vi "MotorTuning.vi"() -> ()   [LabVIEW 2017]
uses:
  <vilib>/Platform/TimedLoop/XDataNode/wakeup.ctl
  <vilib>/Platform/TimedLoop/XDataNode/XDNodeRunTimeDep.lvlib
  <vilib>/Platform/TimedLoop/XDataNode/nitl_modes.ctl
  <vilib>/Platform/TimedLoop/XDataNode/timing_clust.ctl
  <vilib>/Platform/TimedLoop/XDataNode/XDataNode.xnode
  <vilib>/addons/control/pid/NI_PID_pid.lvlib
  <vilib>/addons/control/pid/pid.llb/PID Output Rate Limiter (DBL Array).vi
  typeDef/Modes.ctl
  <vilib>/rvi/interface/nirviReadWriteControl/nirviReadWriteControl.xnode
  <vilib>/Utility/error.llb/Error Cluster From Error Code.vi
  <vilib>/rvi/interface/Simulation/niFpgaSimulationCallBeginRW.vi
  <vilib>/rvi/errors/niLvFpgaAdjustHostInterfaceError.vi
  NiFpgaLv.dll
  subVIs_target/GlobalVariables.vi
  <vilib>/addons/control/pid/pid.llb/PID (DBL).vi
panel:
  in  "?":string="PID_M1.txt"
  in  "FF only once":bool=TRUE
  out "noiseCT":dbl
  in  "amp and freq":dbl[](array[numeric])=[0.0, 0.0, 0.0, 0.0]
  out "nS":dbl
  in  "Noise":bool
  out "dWrite":dbl[](array[numeric])
  in  "filtLowCutFreq":dbl=10.0
  in  "filtOrder":i32=2
  in  "PID_betas":dbl[](array[numeric])=[1.0]
  in  "Mag (N)":dbl=20.0
  in  "Force":bool
  in  "PID gains":T1(array[cluster])=[{"proportional gain (Kc)"=3.5, "integral time (Ti, min)"=0.001, "derivative time (Td, min)"=0.0004}]
  in  "?":bool
  in  "Motor No":i32
  out "currentTension":dbl
  out "whichMotors":i32[](array[numeric])
  out "nMotors":i32
  out "ff+fb OP (N)":dbl[](array[numeric])
  out "setTension":dbl
  out "Period":dbl
  in  "PID_OP_upLim":dbl=60.0
  out "frictionV":dbl[](array[numeric])
  out "CableReelAng(deg)":dbl[](array[numeric])
  out "refnum out":refnum<file>
  in  "Record":bool
  in  "SetPt loop period":i64=4000
  in  "Voltage":dbl(slide) scale=0.0..2.5
  in  "Stop":bool
  in  "pidLpPrd":i64=1000
  in  "Manual":bool
  out "FFnFB OP (N)":dbl[](array[numeric])
  out "Voltage O/P (V)":dbl[](graph)
  out "?":T2(graph)
  in  "?":bool
  in  "freq and step":dbl[](array[numeric])=[0.0, 0.0, 0.0, 0.0]
  in  "Constant":bool
  in  "Idle":bool
  in  "LoadCell No":i32
  out "OP (V)":dbl[](array[numeric])
  out "Iteration Duration":i64
  out "Iteration Duration 2":i64
  # "Amp (N)\n\nfreq (Hz)\n\nSTEP (N)"
  # "Desired (N)"
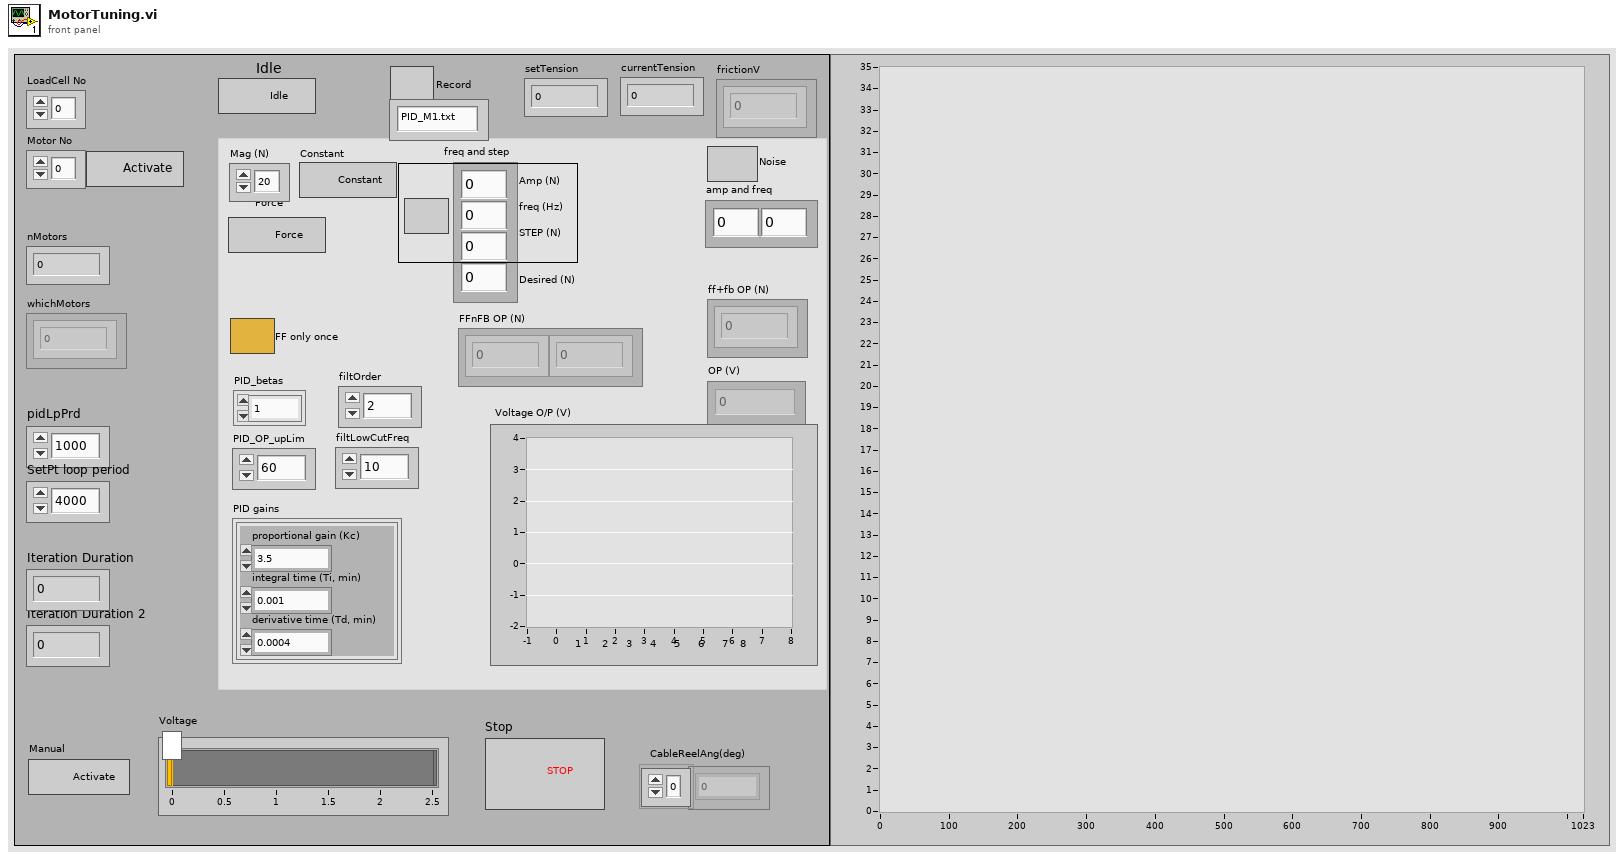
[diagram p1: front panel]
types:
  T1 = cluster{"proportional gain (Kc)":dbl, "integral time (Ti, min)":dbl, "derivative time (Td, min)":dbl}[]
  T2 = cluster{"[0]":dbl, "[1]":dbl, "[2]":dbl, "[3]":dbl, "[4]":dbl, "[5]":dbl, "[6]":dbl, "[7]":dbl}
  T3 = typedef "Modes.ctl" = enum16{"Idle", "Constant", "Force", "Pert"}
  T4 = enum16{"open", "replace", "create", "open or create", "replace or create", "replace or create with confirmation"}
  T5 = typedef "XDNodeRunTimeDep.lvlib/timing_clust.ctl" = cluster{"Expected End [f-1]":u64, "Actual End [f-1]":u64, "Finished Late? [f-1]":bool, "Expected End [i-1]":u64, "Actual End [i-1]":u64, "Finished Late? [i-1]":bool, "Expected Start [i]":u64, "Actual Start [i]":u64, "Expected Start [f]":u64, "Actual Start [f]":u64, "Source Name":string, "Structure Name":string, "Period":i64, "Deadline":i64, "Offset":i64, "Start":i64, "Priority":i32, "Timeout":i32, "Mode":T6, "Wakeup Reason":T7, "Error":errorcluster, "Source Type":string, "Secondary Source Type":string, "Global End Time":u64, "Global Start Time":u64, "Frame Duration":u64, "Iteration Duration":u64, "Assigned CPU":i32, "I/O Scan Engine Mode":u32}
  T6 = typedef "XDNodeRunTimeDep.lvlib/nitl_modes.ctl" = enum32{"No Change", "Process missed periods, maintain original phase", "Discard missed periods, maintain original phase", "Process missed periods, ignore original phase", "Discard missed periods, ignore original phase"}
  T7 = typedef "XDNodeRunTimeDep.lvlib/wakeup.ctl" = enum32{"Normal", "Aborted", "Asynchronous wakeup", "Timing source error", "Timed loop error", "Timeout"}
  T8 = cluster{"fsp":dbl, "fvp":dbl, "fsn":dbl, "fvn":dbl}[]
  T9 = typedef "constants_LL.ctl" = cluster{"zero array":dbl[], "decRate_ff":dbl[], "Motor constants":dbl[], "PID gains":cluster{"proportional gain (Kc)":dbl, "integral time (Ti, min)":dbl, "derivative time (Td, min)":dbl}[], "decRate _fb":dbl[], "PID_OP_upLim":dbl, "nMotors":i32, "PID_betas":dbl[], "filtOrder":i32, "filtLowCutFreq":dbl, "filtSamplFreq":dbl, "whichMotors":i32[], "nMotors 1":i32, "nMotors 2":i32, "Motor constants pel":dbl[], "Motor constants trunk":dbl[]}
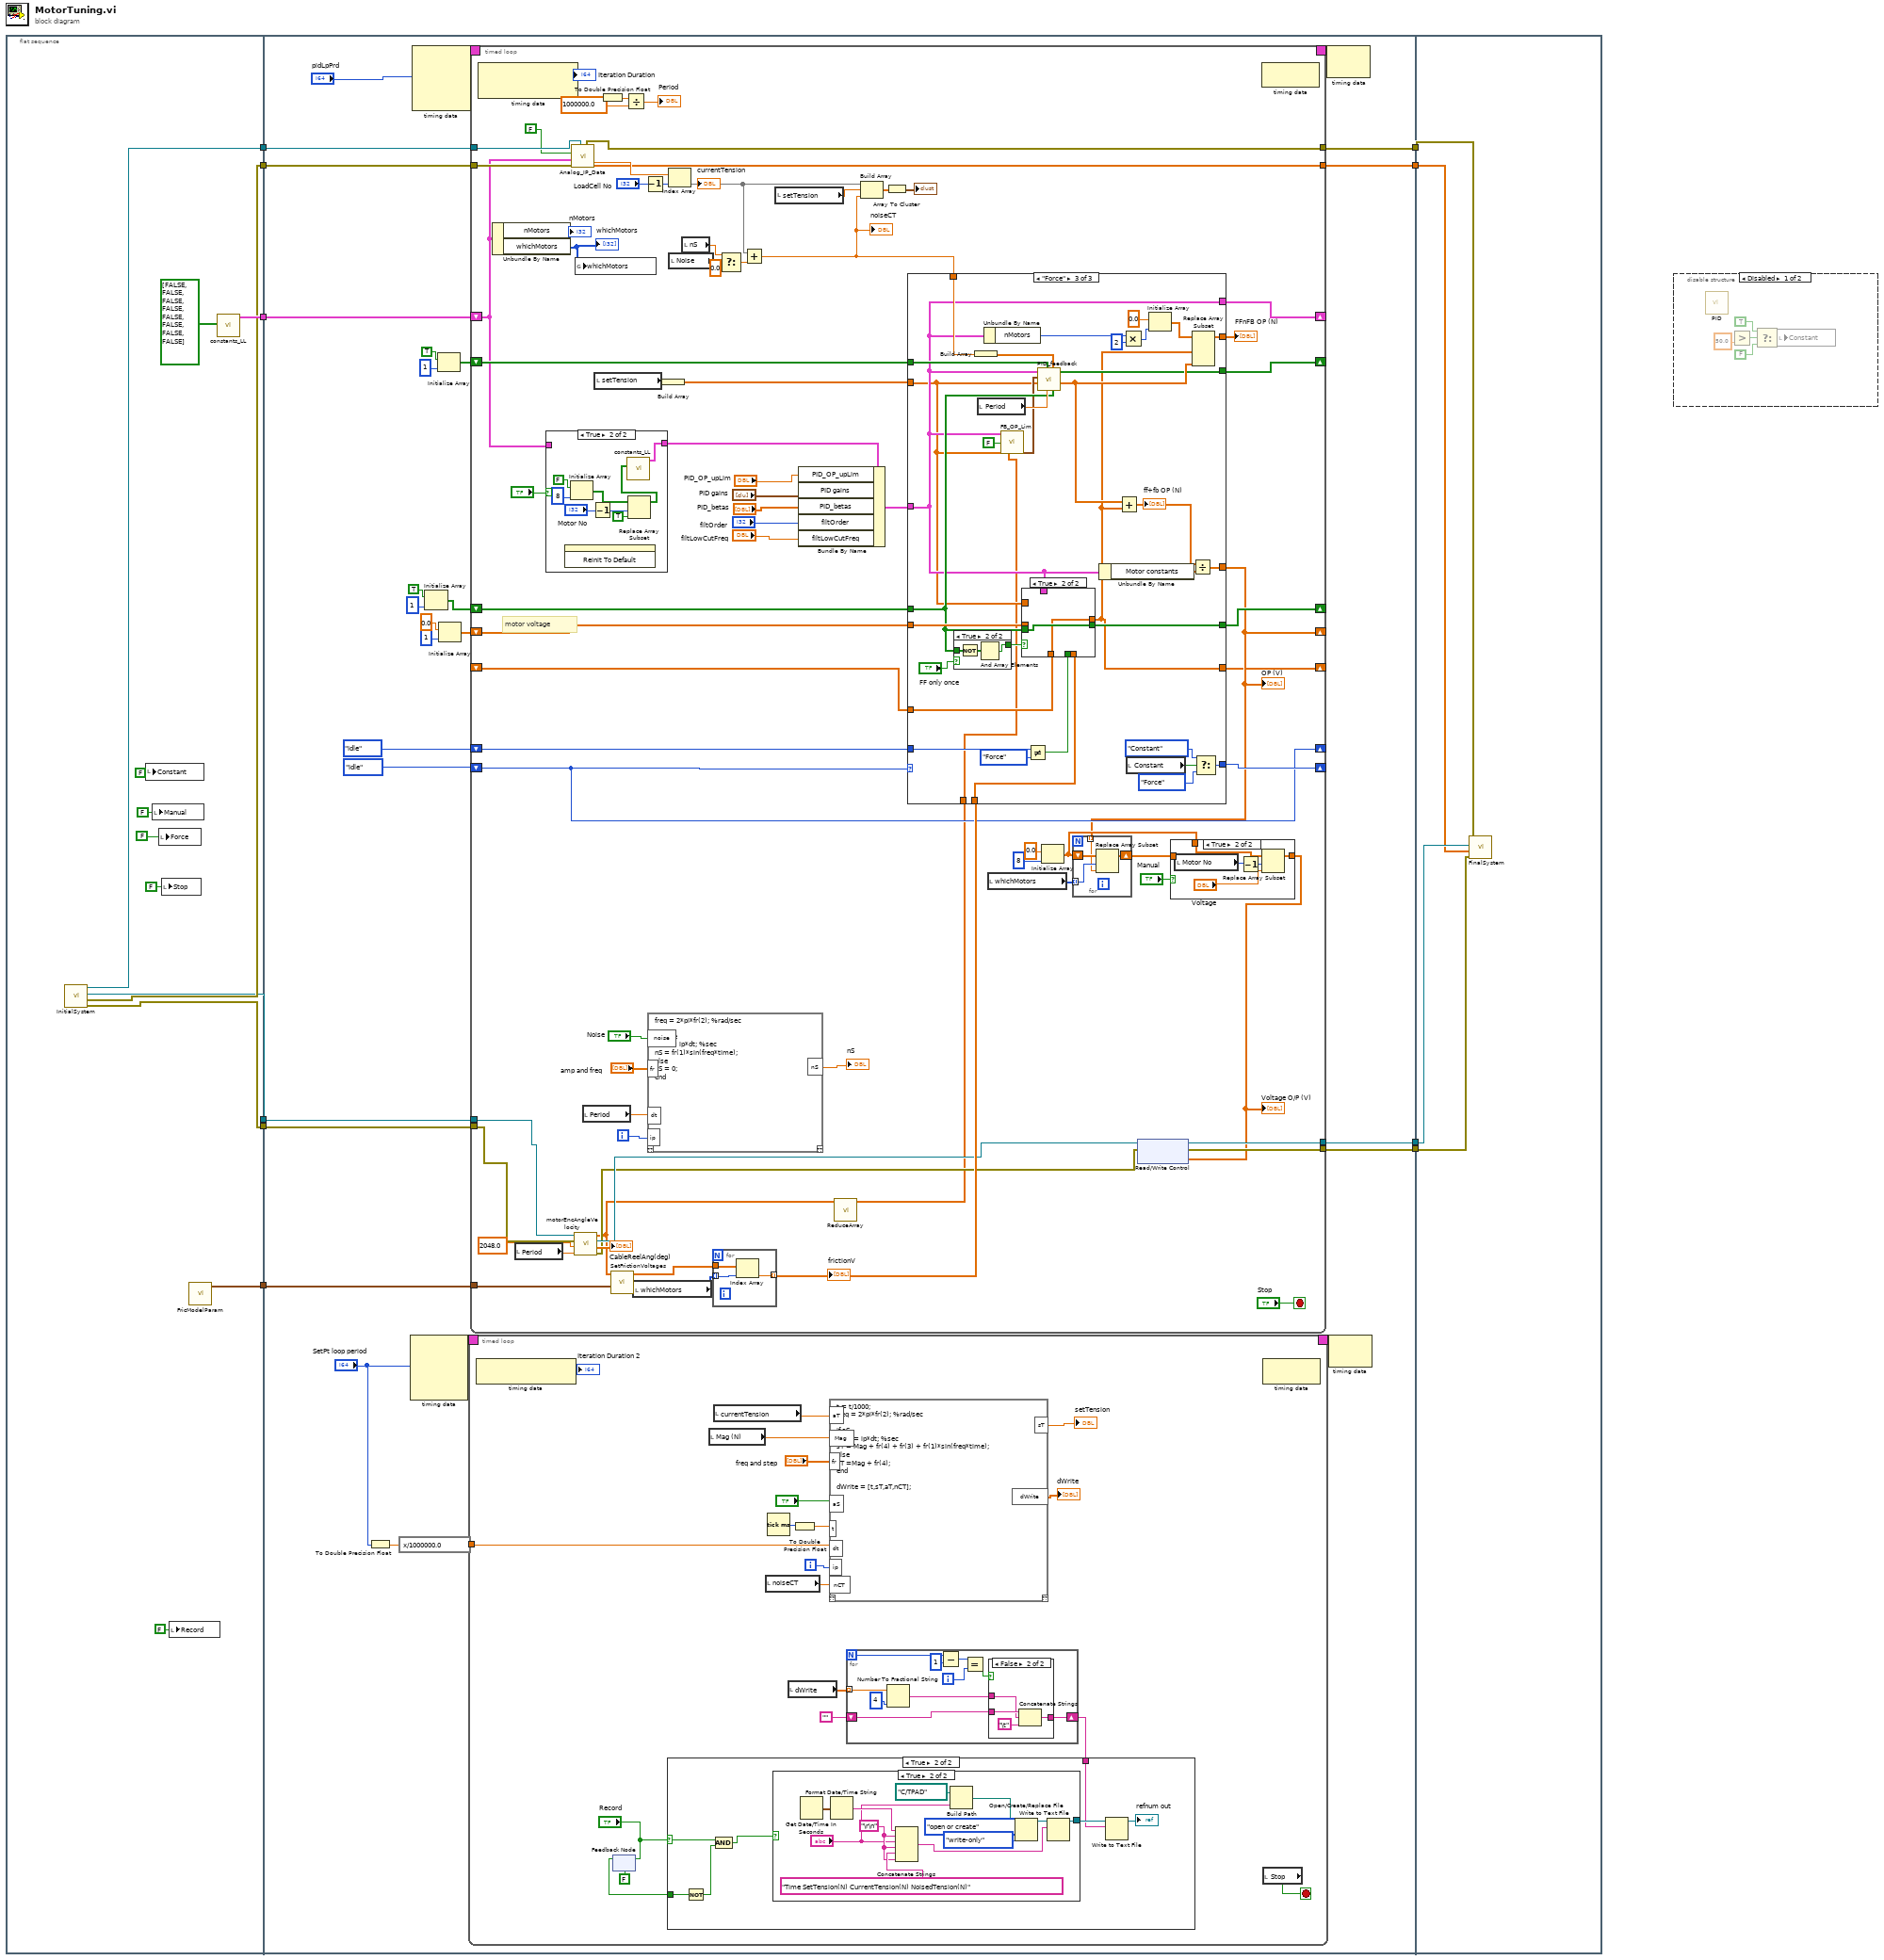
[diagram p0: block diagram]
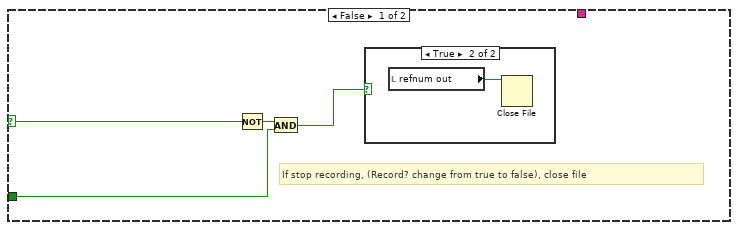
[diagram p3: hidden frame]
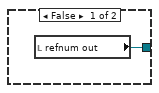
[diagram p5: hidden frame]
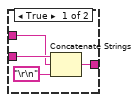
[diagram p6: hidden frame]
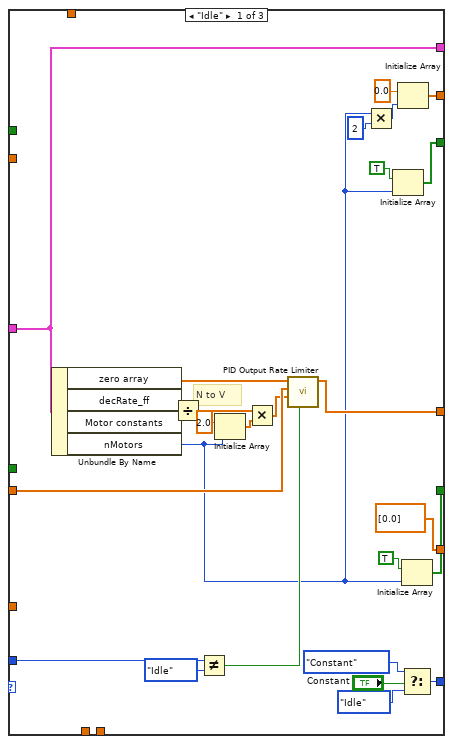
[diagram p9: hidden frame]
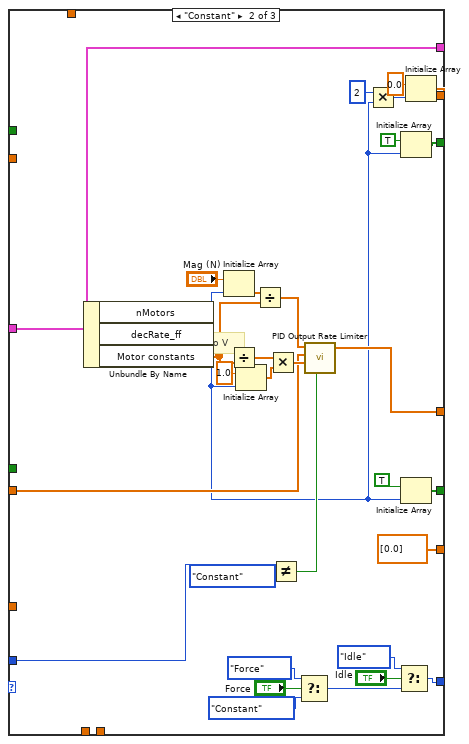
[diagram p10: hidden frame]
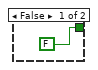
[diagram p11: hidden frame]
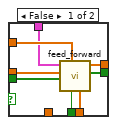
[diagram p12: hidden frame]
diagram:
  n1 = flat-sequence {
    tunnel: [w14] -> w10
    tunnel: [w12] -> w9
    tunnel: [w22] -> w8
    tunnel: [w21] -> w7
    tunnel: [w11] -> w5
    tunnel: [w13] -> w4
    tunnel: w10 -> [w47]
    tunnel: [w46] -> w6
    tunnel: w9 -> [w45]
    tunnel: w8 -> [w44]
    tunnel: w7 -> [w43]
    tunnel: w5 -> [w27]
    tunnel: w4 -> [w26]
    tunnel: [w25] -> w3
    tunnel: [w24] -> w2
    tunnel: [w23] -> w1
    tunnel: w6 -> [w335]
    tunnel: w3 -> [w338]
    tunnel: w2 -> [w337]
    tunnel: w1 -> [w336]
    frame #0 {
      n2 = call "InitialSystem.vi"() -> ("error out"=w13:errorcluster, "error out 2"=w12:errorcluster, "FPGA VI Reference Out"=w11:refnum<k20>, "Refnum out"=w14:refnum<k21>)  [unwired: 8 in]
      n3 = local write "Constant"(FALSE ("Force")) -> ()
      n4 = local write "Manual"(FALSE ("Manual")) -> ()
      n5 = local write "Force"(FALSE ("Force")) -> ()
      n6 = local write "Stop"(FALSE ("Stop")) -> ()
      n7 = local write "Record"(FALSE ("Record")) -> ()
      n8 = call "FricModelParam.vi"() -> ("FricModelParam"=w21:T8)  [unwired: 11 in]
      n9 = call "constants_LL.vi"("MotorsInUse"=bool[] [FALSE, FALSE, FALSE, FALSE, FALSE, FALSE, FALSE, FALSE] ("Enable Motors")) -> ("Constants LL"=w22:T9)  [unwired: 10 in]
    }
    frame #1 {
      n10 = To Double Precision Float(number="SetPt loop period") -> (double precision float=w37:dbl)
      n11 = expression code="x/1000000.0"(w37) -> (w39:dbl)
      n12 = node-c288("SetPt loop period") -> (w49:T5)  [unwired: 3 in]
      n13 = node-c288("pidLpPrd") -> (w51:T5)  [unwired: 3 in]
      n14 = Initialize Array(TRUE, 1 ("dimension size")) -> (w31:bool[])
      n15 = Initialize Array(TRUE, 1 ("dimension size")) -> (w30:bool[])
      n16 = Initialize Array(0.0 ("element"), 1 ("dimension size")) -> (w36:dbl[])
      n17 = timed-loop {
        timing: w49 -> [_]
        timing-out: [_] -> w48
        tunnel: w39 -> [w66]
        i -> [w58]
        stop <- w67 stop-if-true
        n18 = node-c288() -> (→"Iteration Duration 2":i64)  [unwired: 1 in]
        n19 = feedback-in #1("Record") -> ()
        n20 = feedback #1(FALSE) -> (w61:bool)
        n21 = local read "Mag (N)"() -> (w55:dbl)
        n22 = local read "currentTension"() -> (w56:dbl)
        n23 = local read "noiseCT"() -> (w52:dbl)
        n24 = Tick Count (ms)() -> (millisecond timer value=w70:u32)
        n25 = local read "dWrite"() -> (w53:dbl[])
        n26 = To Double Precision Float(number=w70) -> (double precision float=w69:dbl)
        n27 = mathscript code="t = t/1000;\nfreq = 2*pi*fr(2); %rad/sec\n\nif aS\ntime = ip*dt; %sec\nsT = Mag + fr(4) + fr(3) + fr(1)*sin(freq*time);\nelse\nsT =Mag + fr(4);\nend\n\ndWrite = [t,sT,aT,nCT];"("aS"="?", "ip"=w58, "fr"="freq and step", "t"=w69, "aT"=w56, "dt"=w66, "Mag"=w55, "nCT"=w52) -> ("dWrite"=→"dWrite":dbl[], "sT"=→"setTension":dbl)  [unwired: 1 in, 1 out]
        n28 = for {
          N -> [w100]
          tunnel: w53 -> [w104] mode=indexing
          shift-right: [w103] -> w63
          shift-left: "" -> [w102]
          i -> [w97]
          n29 = Number To Fractional String(number=w104, precision (6)=i16 4) -> (F-format string=w101:string)  [unwired: 2 in]
          n30 = Subtract(x=w100, y=1) -> (x-y=w98:i32)
          n31 = Equal?(x=w98, y=w97) -> (x = y?=w96:bool)
          n32 = case shown="False" w96 {
            tunnel: [w109 w113] -> w103
            tunnel: w102 -> [w108 w112]
            tunnel: w101 -> [w107 w111]
            frame True {
              n33 = Concatenate Strings(w108, w107, "\r\n") -> (w109:string)
            }
            frame False {
              n34 = Concatenate Strings(w112, w111, "\t") -> (w113:string)
            }
          }
        }
        n35 = case shown="True" "Record" {
          selector: "Record" -> [w73 w76]
          tunnel: w63 -> [_ w81]
          tunnel: w61 -> [w72 w79]
          frame False {
            # "If stop recording, (Record? change from true to false), close file"
            n36 = Not(x=w73) -> (.not. x?=w74:bool)
            n37 = And(x=w74, y=w72) -> (x .and. y?=w71:bool)
            n38 = case shown="True" w71 {
              frame False {
              }
              frame True {
                n39 = local read "refnum out"() -> (w75:refnum<file>)
                n40 = Close File(refnum=w75) -> ()  [unwired: 1 in, 2 out]
              }
            }
          }
          frame True {
            n41 = Not(x=w79) -> (.not. x?=w78:bool)
            n42 = And(x=w76, y=w78) -> (x .and. y?=w77:bool)
            n43 = case shown="True" w77 {
              tunnel: [w83 w85] -> w82
              frame False {
                n44 = local read "refnum out"() -> (w83:refnum<file>)
              }
              frame True {
                w92 = "\r\n"
                n45 = Get Date/Time In Seconds() -> (seconds since 1Jan1904=w95:timestamp)
                n46 = Format Date/Time String(seconds (now)=w95) -> (date/time string=w94:string)  [unwired: 2 in]
                n47 = Concatenate Strings(w94, w92, "?", w92, "Time SetTension(N) CurrentTension(N) NoisedTension(N)", w92) -> (w86:string)
                n48 = Build Path(base path=path "C:/TPAD", name or relative path="?") -> (appended path=w90:path)
                n49 = Open/Create/Replace File(file path (use dialog)=w90, operation (0:open)=T4."open or create", access (0:read/write)=enum16{"read/write", "read-only", "write-only"}."write-only") -> (refnum out=w87:refnum<file>)  [unwired: 3 in, 2 out]
                n50 = Write to Text File(file (use dialog)=w87, text=w86) -> (refnum out=w85:refnum<file>)  [unwired: 2 in, 2 out]
              }
            }
            n51 = Write to Text File(file (use dialog)=w82, text=w81) -> (refnum out=→"refnum out":refnum<file>)  [unwired: 2 in, 2 out]
          }
        }
        n52 = node-c288() -> ()  [unwired: 1 in, 1 out]
        n53 = local read "Stop"() -> (w67:bool)
      }
      n54 = timed-loop {
        timing: w51 -> [_]
        timing-out: [_] -> w50
        tunnel: w47 -> [w135]
        tunnel: [w134] -> w46
        tunnel: w45 -> [w196]
        shift-right: [w158] -> _
        shift-left: Modes."Idle" ("Enum") -> [w195]
        shift-right: [w194] -> _
        shift-left: Modes."Idle" ("Enum") -> [w158]
        shift-right: [w157] -> _
        shift-left: w36 -> [w189]
        tunnel: w43 -> [w193]
        shift-right: [w191] -> _
        shift-left: w31 -> [w190]
        shift-right: [w183] -> _
        shift-left: w30 -> [w184]
        shift-right: [w165] -> _
        shift-left: w44 -> [w136]
        shift-right: [w149] -> _
        shift-left: _ -> [w148]
        tunnel: w27 -> [w129]
        tunnel: w26 -> [w128]
        tunnel: [w131] -> w25
        tunnel: [w130] -> w24
        tunnel: [w124] -> w23
        i -> [w141]
        stop <- "Stop" stop-if-true
        # "motor voltage"
        n55 = node-c288() -> (→"Iteration Duration":i64, w178:i64)  [unwired: 1 in]
        n56 = Unbundle By Name(w136) -> ("nMotors"=→"nMotors":i32, "whichMotors"=w122:i32[])
        "whichMotors" <- w122
        n57 = local read "Period"() -> (w176:dbl)
        n58 = case shown="True" "?" {
          tunnel: [w207 w210] -> w151
          tunnel: w136 -> [w207 _]
          frame False {
          }
          frame True {
            n59 = invoke class="Bool (strict)" method="Reinit To Default"() -> ()  [unwired: 3 in, 3 out]
            n60 = Initialize Array(FALSE, 8 ("dimension size")) -> (w213:bool[])
            n61 = Decrement(x="Motor No") -> (x-1=w208:i32)
            n62 = Replace Array Subset(array=w213, new element=TRUE ("new element/subarray"), index=w208) -> (w211:bool[])
            n63 = call "constants_LL.vi"("MotorsInUse"=w211) -> ("Constants LL"=w210:T9)  [unwired: 10 in]
          }
        }
        n64 = call "Analog_IP_Data.vi"("Refnum in"=w135, "error in (no error)"=w196, "Constants LL"=w136, "Use ATI"=FALSE ("ATI Connected")) -> ("Tared FT Reading"=w124:dbl[], "Toe"=w132:dbl, "error out"=w134:errorcluster)  [unwired: 1 in, 4 out]
        n65 = call "motorEncAngleVelocity.vi"("dt"=w176, "CPR"=2048.0, "error in (no error)"=w128, "Refnum in"=w129) -> ("error out"=w126:errorcluster, "CableReelPos(deg)"=→"CableReelAng(deg)":dbl[], "Refnum out"=w127:refnum<k20>, "CableReelVel(RPM)"=w123:dbl[])  [unwired: 4 in]
        n66 = global write "GlobalVariables.vi" "whichMotors"(w122) -> ()
        n67 = local read "Period"() -> (w138:dbl)
        n68 = local read "setTension"() -> (w173:dbl)
        n69 = To Double Precision Float(number=w178) -> (double precision float=w180:dbl)
        n70 = call "SetFrictionVoltages.vi"("FricModelParam"=w193, "EncoderVelocity(RPM)"=w123) -> ("FrictionVoltages"=w171:dbl[])  [unwired: 9 in]
        n71 = Divide(x=w180, y=1000000.0) -> (x/y=→"Period":dbl)
        n72 = local read "whichMotors"() -> (w170:i32[])
        n73 = Decrement(x="LoadCell No") -> (x-1=w166:i32)
        n74 = mathscript code="freq = 2*pi*fr(2); %rad/sec\n\nif noise\ntime = ip*dt; %sec\nnS = fr(1)*sin(freq*time);\nelse\nnS = 0;\nend"("ip"=w141, "noise"="Noise", "dt"=w138, "fr"="amp and freq") -> ("nS"=→"nS":dbl)  [unwired: 1 in, 1 out]
        n75 = Build Array(w173) -> (w174:dbl[])
        n76 = Index Array(array=w132, index=w166) -> (element=w143)
        "currentTension" <- w143
        n77 = local read "Noise"() -> (w147:bool)
        n78 = local read "nS"() -> (w146:dbl)
        n79 = for {
          tunnel: w170 -> [w217] mode=indexing
          tunnel: w171 -> [w218]
          tunnel: [w216] -> w169 mode=indexing
          n80 = Index Array(array=w218, index=w217) -> (element=w216:dbl)
        }
        "frictionV" <- w169
        n81 = Select(t=w146, s=w147, f=0.0) -> (s? t:f=w144:dbl)
        n82 = Add(x=w143, y=w144) -> (x+y=w142:dbl)
        "noiseCT" <- w142
        n83 = local read "setTension"() -> (w175:dbl)
        n84 = Bundle By Name(cluster=w151, "PID_OP_upLim"="PID_OP_upLim", "PID gains"="PID gains", "PID_betas"="PID_betas", "filtOrder"="filtOrder", "filtLowCutFreq"="filtLowCutFreq") -> (w150:T9)
        n85 = call "ReduceArray.vi"("I/P Array"=w123) -> ("Reduced Array"=w121:dbl[])  [unwired: 10 in]
        n86 = Build Array(w143, w175, w142) -> (w187:dbl[])
        n87 = Array To Cluster(array=w187) -> (cluster=→"?":T2)
        n88 = case shown="\"Force\"" w158 {
          tunnel: [w222 w273 w290] -> w194
          tunnel: w195 -> [w245 w271 w312]
          tunnel: [w238 w258 w303] -> w157
          tunnel: w189 -> [w243 w253 w309]
          tunnel: w142 -> [_ _ w285]
          tunnel: w169 -> [_ _ w299]
          tunnel: [w231 w257 w300] -> w191
          tunnel: w190 -> [_ _ w289]
          tunnel: w174 -> [_ _ w279]
          tunnel: [w235 w259 w311] -> w188
          tunnel: w184 -> [_ _ w302]
          tunnel: [w233 w260 w301] -> w183
          tunnel: w150 -> [w230 w251 w282]
          tunnel: [w230 w251 w282] -> w165
          tunnel: [dbl[] [0.0] ("ff output") dbl[] [0.0] ("ff output") w287] -> w149
          tunnel: w148 -> [_ _ w286]
          tunnel: w121 -> [_ _ w278]
          frame "Idle" {
            # "N to V"
            n89 = Unbundle By Name(w230) -> ("zero array"=w240:dbl[], "decRate_ff"=w239:dbl[], "Motor constants"=w237:dbl[], "nMotors"=w226:i32)
            n90 = Divide(x=w239, y=w237) -> (x/y=w242:dbl[])
            n91 = Not Equal?(x=w245, y=Modes."Idle" ("Enum")) -> (x != y?=w244:bool)
            n92 = Initialize Array(2.0 ("element"), w226) -> (w228:dbl[])
            n93 = Multiply(x=w242, y=w228) -> (x*y=w241:dbl[])
            n94 = call-poly <vilib>:"PID Output Rate Limiter.vi"("reinitialize? (F)"=w244, "output rate (EGU/min)"=w241, "initial output"=w243, "input (controller output)"=w240) -> ("output"=w238:dbl[])  [unwired: 4 in, 1 out]
            n95 = Multiply(x=w226, y=2 ("dimension size")) -> (x*y=w225:i32)
            n96 = Initialize Array(TRUE, w226) -> (w233:bool[])
            n97 = Initialize Array(0.0 ("element"), w225) -> (w235:dbl[])
            n98 = Initialize Array(TRUE, w226) -> (w231:bool[])
            n99 = Select(t=Modes."Constant" ("Enum"), s="Constant", f=Modes."Idle" ("Enum")) -> (s? t:f=w222:T3)
          }
          frame "Constant" {
            # "N to V"
            n100 = Unbundle By Name(w251) -> ("nMotors"=w249:i32, "decRate_ff"=w256:dbl[], "Motor constants"=w255:dbl[])
            n101 = Initialize Array("Mag (N)", w249) -> (w270:dbl[])
            n102 = Divide(x=w256, y=w255) -> (x/y=w266:dbl[])
            n103 = Initialize Array(1.0 ("element"), w249) -> (w269:dbl[])
            n104 = Divide(x=w270, y=w255) -> (x/y=w254:dbl[])
            n105 = Multiply(x=w266, y=w269) -> (x*y=w267:dbl[])
            n106 = Not Equal?(x=w271, y=Modes."Constant" ("Enum")) -> (x != y?=w252:bool)
            n107 = Select(t=Modes."Force" ("Enum"), s="Force", f=Modes."Constant" ("Enum")) -> (s? t:f=w275:T3)
            n108 = call-poly <vilib>:"PID Output Rate Limiter.vi"("reinitialize? (F)"=w252, "output rate (EGU/min)"=w267, "initial output"=w253, "input (controller output)"=w254) -> ("output"=w258:dbl[])  [unwired: 4 in, 1 out]
            n109 = Multiply(x=2, y=w249) -> (x*y=w262:i32)
            n110 = Select(t=Modes."Idle" ("Enum"), s="Idle", f=w275) -> (s? t:f=w273:T3)
            n111 = Initialize Array(TRUE, w249) -> (w260:bool[])
            n112 = Initialize Array(TRUE, w249) -> (w257:bool[])
            n113 = Initialize Array(0.0 ("element"), w262) -> (w259:dbl[])
          }
          frame "Force" {
            n114 = case shown="True" "FF only once" {
              tunnel: w289 -> [_ w315]
              tunnel: [FALSE w314] -> w288
              frame False {
              }
              frame True {
                n115 = Not(x=w315) -> (.not. x?=w316:bool[])
                n116 = And Array Elements(Boolean array=w316) -> (logical AND=w314:bool)
              }
            }
            n117 = Build Array(w285) -> (w307:dbl[])
            n118 = local read "Period"() -> (w306:dbl)
            n119 = Unbundle By Name(w282) -> ("nMotors"=w294:i32)
            n120 = call "FB_OP_Lim.vi"("Constants LL"=w282, "WirePullComp"=FALSE, "SetTension"=w279, "vel (rpm)"=w278) -> ("PID_OP_Lim"=w281:cluster{"PID_OP_upLim":dbl, dbl}[])  [unwired: 11 in]
            n121 = Not Equal?(x=w312, y=Modes."Force" ("Enum")) -> (x != y?=w308:bool)
            n122 = case shown="True" w288 {
              tunnel: w309 -> [w324 _]
              tunnel: w308 -> [w323 _]
              tunnel: [w322 w325] -> w287
              tunnel: [w321 w326] -> w300
              tunnel: w279 -> [w320 _]
              tunnel: w299 -> [w319 _]
              tunnel: w282 -> [w318 _]
              tunnel: w289 -> [w317 w326]
              tunnel: w286 -> [_ w325]
              frame False {
                n123 = call "feed_forward.vi"("fricCompV"=w319, "reinitialize"=w323, "SetTension"=w320, "limit logic in"=w317, "preMotorV"=w324, "Constants LL"=w318) -> ("limit logic out"=w321:bool[], "ff output"=w322:dbl[])  [unwired: 4 in]
              }
              frame True {
              }
            }
            n124 = call "PID_feedback.vi"("Reintialize"=w289, "currentT"=w307, "dt (s)"=w306, "LimitLogicIn"=w302, "SetTension"=w279, "PID_OP_Lim"=w281, "Constants LL"=w282) -> ("pidOP"=w304:dbl[], "limit logic out"=w301:bool[])  [unwired: 3 in]
            n125 = Unbundle By Name(w282) -> ("Motor constants"=w305:dbl[])
            n126 = Add(x=w304, y=w287) -> (x+y=w310:dbl[])
            "ff+fb OP (N)" <- w310
            n127 = Multiply(x=w294, y=2 ("dimension size")) -> (x*y=w296:i32)
            n128 = local read "Constant"() -> (w283:bool)
            n129 = Initialize Array(0.0 ("element"), w296) -> (w295:dbl[])
            n130 = Divide(x=w310, y=w305) -> (x/y=w303:dbl[])
            n131 = Replace Array Subset(array=w295, new element #1=w287, new element #2=w304) -> (w311:dbl[])  [unwired: 2 in]
            n132 = Select(t=Modes."Constant" ("Enum"), s=w283, f=Modes."Force" ("Enum")) -> (s? t:f=w290:T3)
          }
        }
        "OP (V)" <- w157
        "FFnFB OP (N)" <- w188
        n133 = local read "whichMotors"() -> (w159:i32[])
        n134 = Initialize Array(0.0 ("element"), 8 ("dimension size")) -> (w160:dbl[])
        n135 = for {
          tunnel: w159 -> [w200] mode=indexing
          tunnel: w157 -> [w197] mode=indexing
          shift-right: [w199] -> w164
          shift-left: w160 -> [w198]
          n136 = Replace Array Subset(array=w198, new element=w197, index=w200) -> (w199:dbl[])
        }
        n137 = case shown="True" "Manual" {
          tunnel: w164 -> [w201 _]
          tunnel: [w201 w206] -> w125
          tunnel: w160 -> [_ w204]
          frame False {
          }
          frame True {
            n138 = local read "Motor No"() -> (w202:i32)
            n139 = Decrement(x=w202) -> (x-1=w205:i32)
            n140 = Replace Array Subset(array=w204, new element="Voltage", index=w205) -> (w206:dbl[])
          }
        }
        "Voltage O/P (V)" <- w125
        n141 = xnode "Read/Write Control"("FPGA VI Reference In"=w127, "error in"=w126, "AO_Value"=w125) -> ("FPGA VI Reference Out"=w131:refnum<k20>, "error out"=w130:errorcluster)
        n142 = node-c288() -> ()  [unwired: 1 in, 1 out]
      }
      n143 = node-c288(w50) -> ()  [unwired: 1 out]
      n144 = node-c288(w48) -> ()  [unwired: 1 out]
    }
    frame #2 {
      n145 = call "FinalSystem.vi"("error in (no error)"=w337, "error in"=w336, "FPGA VI Reference Out"=w338, "Refnum in"=w335) -> ()  [unwired: 8 in]
    }
  }
  n146 = disable-structure shown="Disabled" {
    frame Disabled {
      n147 = call-poly <vilib>:"PID.vi"() -> ()  [unwired: 10 in, 2 out]
      n148 = Greater?(y=50.0) -> (x=w339:dbl, 0:w343:bool)
      n149 = Select(t=TRUE ("Constant"), s=w343, f=FALSE ("Constant")) -> (s? t:f=w341:bool)
      n150 = local write "Constant"(w341) -> ()
    }
    frame Enabled {
    }
  }
